vi "Read from File.vi"(8 "error in (no error)":errorcluster, 10 "INI Ref":T1, 11 "Timing Action in":refnum<class "Timing Action.lvclass">) -> (0 "error out":errorcluster, 2 "INI Ref out":T1, 3 "Timing Action out":refnum<class "Timing Action.lvclass">)   [LabVIEW 2020, in "MacroAssert.lvlib" / "Timing Action.lvclass"]
doc: "Reads associated parameters from the file identified by <B>INI Ref</B>."
uses:
  Timing Action.lvclass
  C:/Users/User/Documents/LabVIEW Data/Projects/MacroAssert/source/Classes/Step/Step.lvclass
  <vilib>/Utility/config.llb/Config Data RefNum.ctl
  Timing Action Type.ctl
  Time Unit.ctl
  <vilib>/Utility/error.llb/Error Cluster From Error Code.vi
  <vilib>/Utility/config.llb/Read Key (String).vi
  <vilib>/Utility/config.llb/Read Key (Double).vi
  Action Step/Action Step.lvclass
  MacroAssert.lvlib
  <vilib>/Utility/config.llb/NI_LVConfig.lvlib
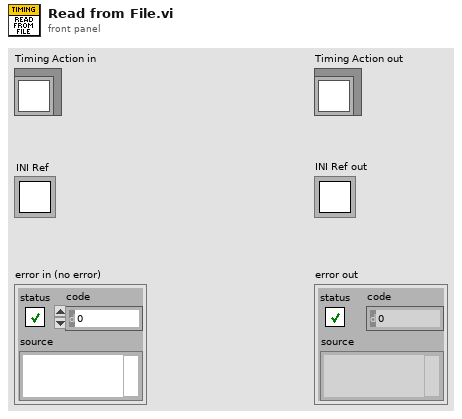
[diagram p1: front panel]
types:
  T1 = typedef "NI_LVConfig.lvlib/Config Data RefNum.ctl" = refnum<k1>
  T2 = typedef "MacroAssert.lvlib/Timing Action.lvclass/Timing Action Type.ctl" = enum16{"Wait", "Wait Until"}
  T3 = typedef "MacroAssert.lvlib/Timing Action.lvclass/Time Unit.ctl" = enum16{"milliseconds", "seconds", "minutes"}
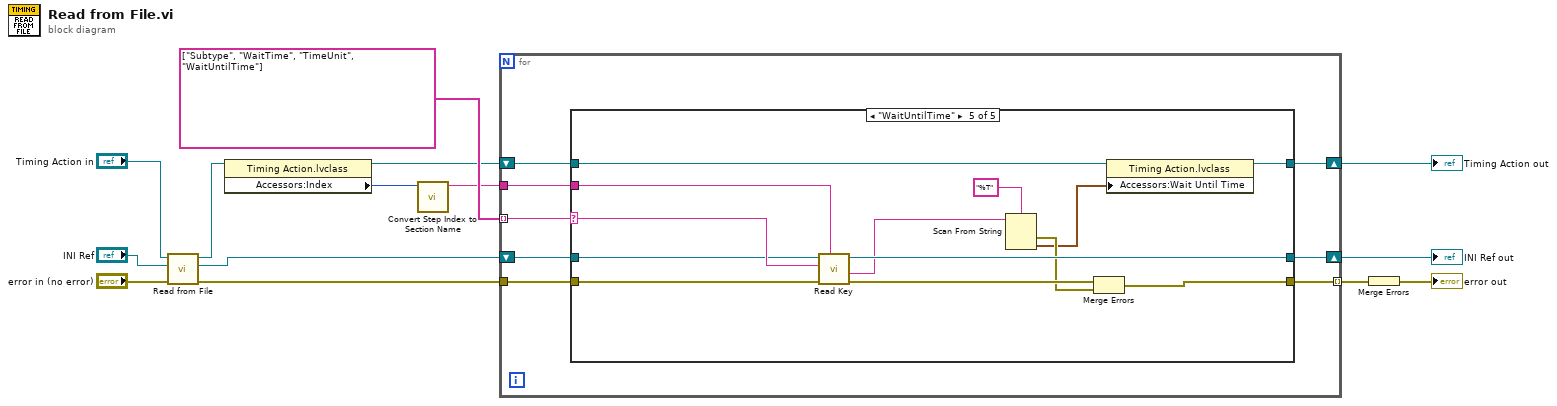
[diagram p0: block diagram]
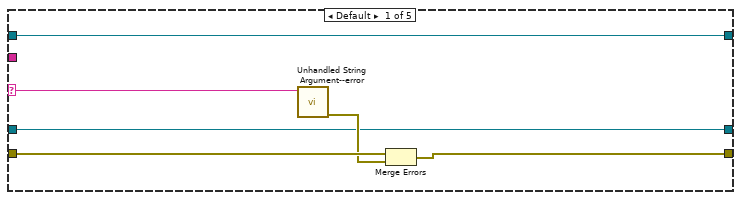
[diagram p2: hidden frame]
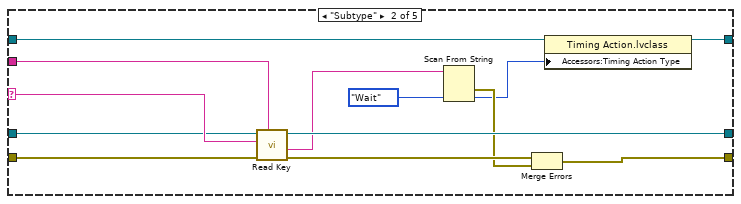
[diagram p3: hidden frame]
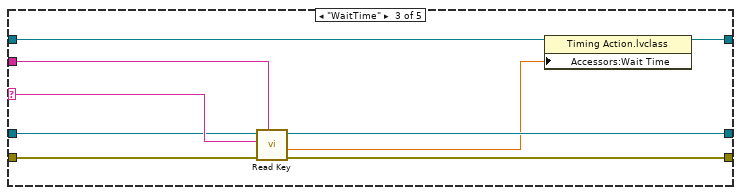
[diagram p4: hidden frame]
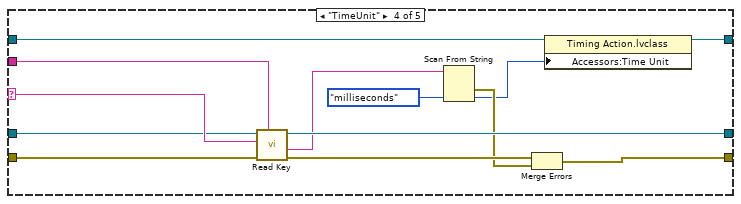
[diagram p5: hidden frame]
diagram:
  n1 = call-parent "Read from File.vi"("error in (no error)"="error in (no error)", "INI Ref"="INI Ref", "Step in"="Timing Action in") -> ("error out"=w11:errorcluster, "INI Ref out"=w8:T1, "Step out"=w14:refnum<class "Timing Action.lvclass">)  [unwired: 6 in]
  n2 = property class="Timing Action.lvclass"(reference=w14) -> (reference out=w9:refnum<class "Timing Action.lvclass">, "Accessors:Index"=w13:i32)  [unwired: 1 in, 1 out]
  n3 = call "Convert Step Index to Section Name.vi"("Step Index"=w13) -> ("Section Name"=w10:string)  [unwired: 10 in]
  n4 = for {
    tunnel: string[] ["Subtype", "WaitTime", "TimeUnit", "WaitUntilTime"] -> [w22] mode=indexing
    tunnel: w11 -> [w21]
    tunnel: w10 -> [w20]
    shift-right: [w18] -> w1
    shift-left: w9 -> [w19]
    tunnel: [w17] -> w7 mode=indexing
    shift-right: [w15] -> w4
    shift-left: w8 -> [w16]
    n5 = case shown="\"WaitUntilTime\"" w22 {
      selector: w22 -> [w25 w36 w45 w58 w71]
      tunnel: w21 -> [w27 w41 w50 w63 w76]
      tunnel: w20 -> [_ w40 w49 w62 w75]
      tunnel: w19 -> [w28 w39 w48 w61 w74]
      tunnel: [w28 w38 w47 w60 w73] -> w18
      tunnel: [w24 w32 w46 w54 w67] -> w17
      tunnel: w16 -> [w23 w35 w44 w57 w70]
      tunnel: [w23 w34 w43 w56 w69] -> w15
      frame Default {
        n6 = call "Unhandled String Argument--error.vi"("Argument"=w25) -> ("error out"=w26:errorcluster)  [unwired: 10 in]
        n7 = Merge Errors(w27, w26) -> (w24:errorcluster)
      }
      frame "Subtype" {
        n8 = call-poly <vilib>:"Read Key.vi"("section"=w40, "error in (no error)"=w41, "key"=w36, "refnum"=w35) -> ("error out"=w37:errorcluster, "value"=w33:string, "refnum out"=w34:T1)  [unwired: 4 in, 1 out]
        n9 = Scan From String(input string=w33, default 1=Timing_Action_Type."Wait" ("Timing Action Type")) -> (error out=w31:errorcluster, output 1=w30:T2)  [unwired: 3 in, 2 out]
        n10 = Merge Errors(w37, w31) -> (w32:errorcluster)
        n11 = property class="Timing Action.lvclass"(reference=w39, "Accessors:Timing Action Type"=w30) -> (reference out=w38:refnum<class "Timing Action.lvclass">)  [unwired: 1 in, 1 out]
      }
      frame "WaitTime" {
        n12 = call-poly <vilib>:"Read Key.vi"("section"=w49, "error in (no error)"=w50, "key"=w45, "refnum"=w44) -> ("error out"=w46:errorcluster, "value"=w42:dbl, "refnum out"=w43:T1)  [unwired: 4 in, 1 out]
        n13 = property class="Timing Action.lvclass"(reference=w48, "Accessors:Wait Time"=w42) -> (reference out=w47:refnum<class "Timing Action.lvclass">)  [unwired: 1 in, 1 out]
      }
      frame "TimeUnit" {
        n14 = call-poly <vilib>:"Read Key.vi"("section"=w62, "error in (no error)"=w63, "key"=w58, "refnum"=w57) -> ("error out"=w59:errorcluster, "value"=w55:string, "refnum out"=w56:T1)  [unwired: 4 in, 1 out]
        n15 = Scan From String(input string=w55, default 1=Time_Unit."milliseconds" ("Time Unit")) -> (error out=w53:errorcluster, output 1=w52:T3)  [unwired: 3 in, 2 out]
        n16 = Merge Errors(w59, w53) -> (w54:errorcluster)
        n17 = property class="Timing Action.lvclass"(reference=w61, "Accessors:Time Unit"=w52) -> (reference out=w60:refnum<class "Timing Action.lvclass">)  [unwired: 1 in, 1 out]
      }
      frame "WaitUntilTime" {
        n18 = call-poly <vilib>:"Read Key.vi"("section"=w75, "error in (no error)"=w76, "key"=w71, "refnum"=w70) -> ("error out"=w72:errorcluster, "value"=w68:string, "refnum out"=w69:T1)  [unwired: 4 in, 1 out]
        n19 = Scan From String(format string="%T", input string=w68) -> (error out=w66:errorcluster, output 1=w64:timestamp)  [unwired: 3 in, 2 out]
        n20 = Merge Errors(w72, w66) -> (w67:errorcluster)
        n21 = property class="Timing Action.lvclass"(reference=w74, "Accessors:Wait Until Time"=w64) -> (reference out=w73:refnum<class "Timing Action.lvclass">)  [unwired: 1 in, 1 out]
      }
    }
  }
  "Timing Action out" <- w1
  "INI Ref out" <- w4
  n22 = Merge Errors(w7) -> (→"error out":errorcluster)
